vi "TelemetryServer.vi"() -> ()   [LabVIEW 2009]
uses:
  Api/TelemetryServer/TelemetryServer_Global.vi
  Instance           7 23Saved   TelemetryServer .vi
panel:
  in  "PROCESS":string="TELEMETRYSERVER"
  out "Counts":u32[](array[numeric])
  out "ID":u32
  in  "ServerName":string="RTC21Summit.Telemetry.Default"
  in  "Channels":string[](array[string])=["FringeTracker[0].CompleteControllerSet.ControllerData.ChannelData[0].CalibratedBinData[0]", "FringeTracker[0].CompleteControllerSet.ControllerData.DLPosition", "StarTracker[1].CompleteControllerSet.KatControllerData.Intensity", "StarTracker[1].CompleteControllerSet.KatControllerData.PeakIntensity", "StarTracker[1].CompleteControllerSet.KatControllerData.FsmX", "StarTracker[1].CompleteControllerSet.KatControllerData.FsmY", "StarTracker[1].CompleteControllerSet.KatControllerData.PointVectorX", "StarTracker[1].CompleteControllerSet.KatControllerData.PointVectorY", "StarTracker[2].CompleteControllerSet.KatControllerData.Intensity", "StarTracker[2].CompleteControllerSet.KatControllerData.PeakIntensity", "StarTracker[2].CompleteControllerSet.KatControllerData.FsmX", "StarTracker[2].CompleteControllerSet.KatControllerData.FsmY", "StarTracker[2].CompleteControllerSet.KatControllerData.PointVectorX", "StarTracker[2].CompleteControllerSet.KatControllerData.PointVectorY", "StarTracker[3].CompleteControllerSet.KatControllerData.Intensity", "StarTracker[4].CompleteControllerSet.KatControllerData.Intensity", "DelayLine[1].CompleteControllerSet.ControllerData.LaserPositionOPD"]
  out "Count":i32(knob)=17 scale=0.0..34.0
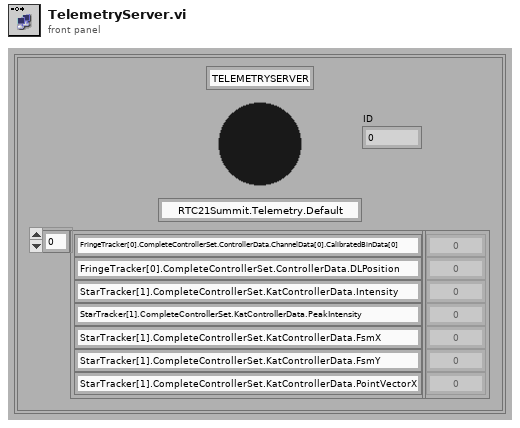
[diagram p1: front panel]
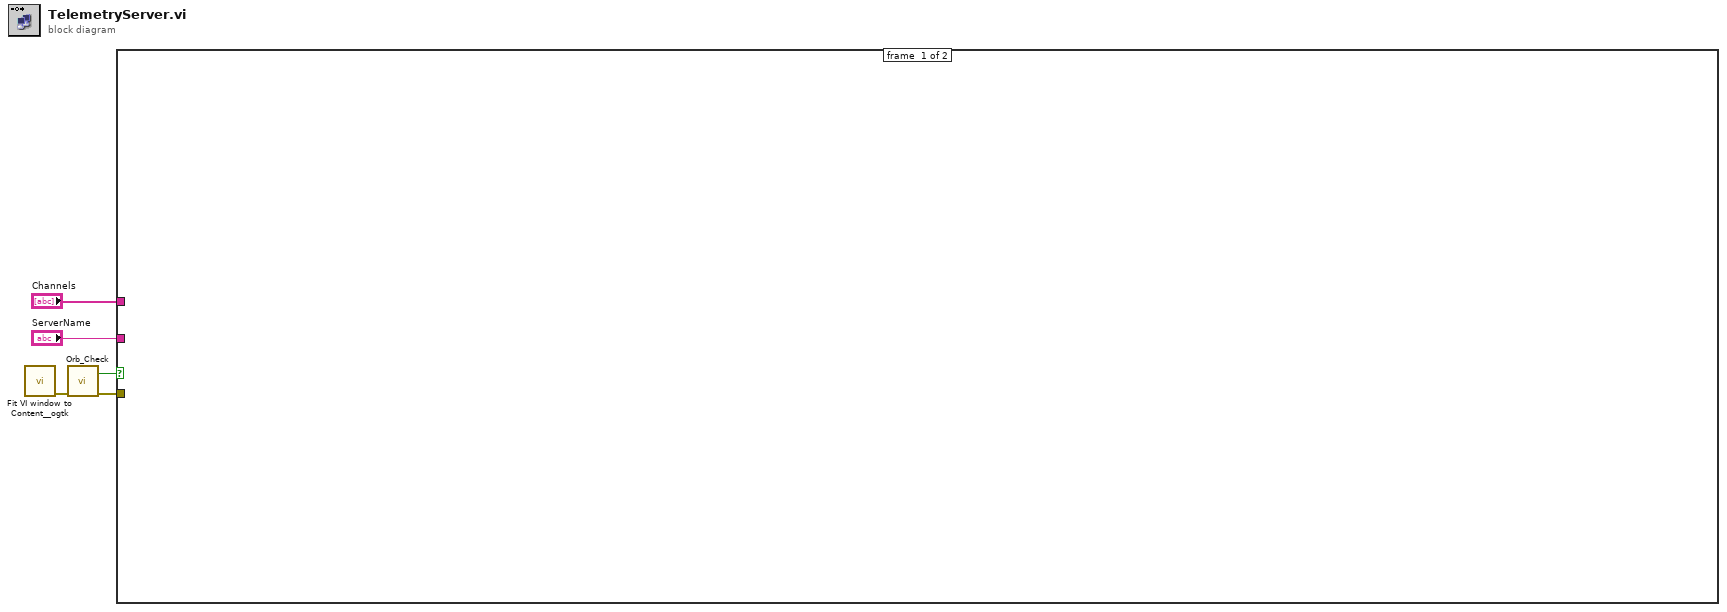
[diagram p0: block diagram]
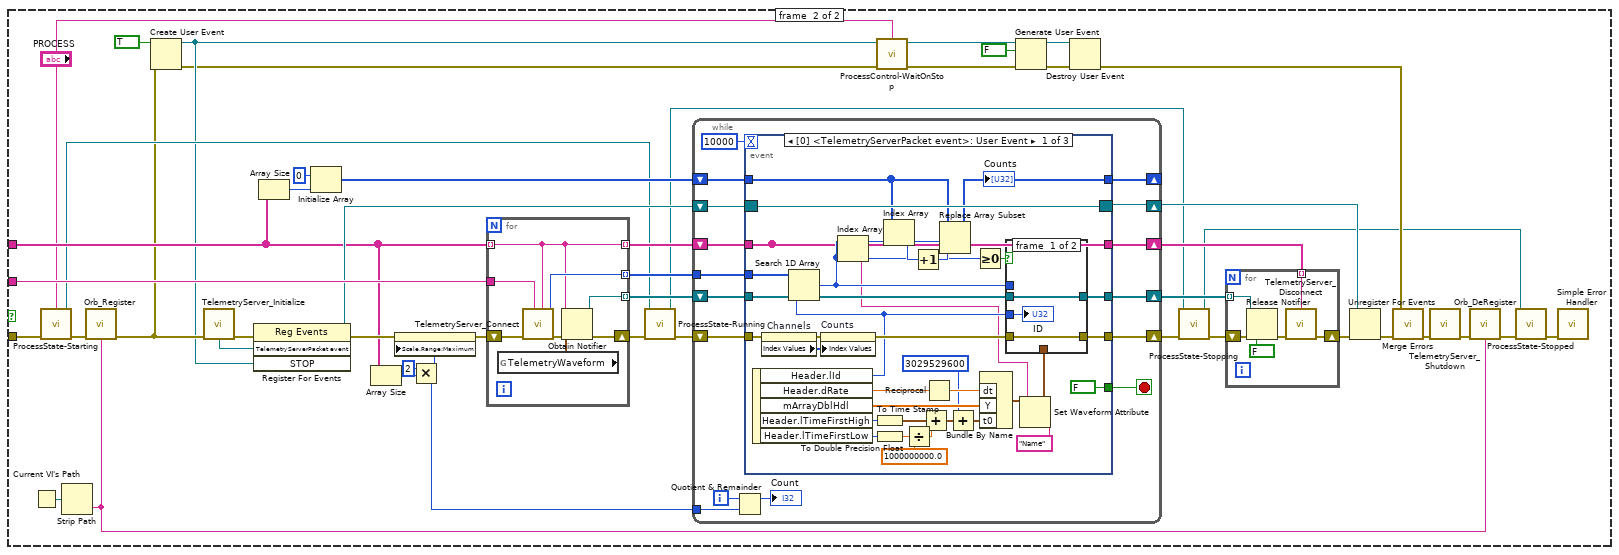
[diagram p2: hidden frame]
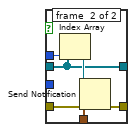
[diagram p3: hidden frame]
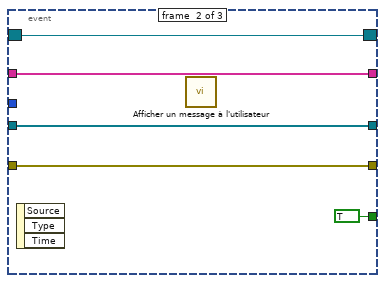
[diagram p4: hidden frame]
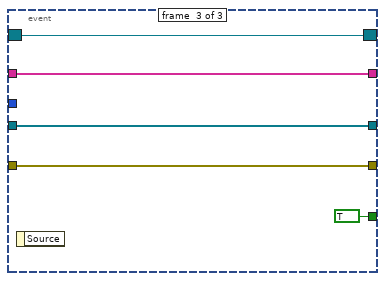
[diagram p5: hidden frame]
diagram:
  n1 = call <userlib>:"Fit VI window to Content__ogtk.vi"() -> ("error out"=w1:errorcluster)  [unwired: 3 in, 4 out]
  n2 = call "Orb_Check.vi"("error in (no error)"=w1) -> ("error out"=w5:errorcluster, "Orb Running ?"=w4:bool)  [unwired: 4 out]
  n3 = case shown="True" w4 {
    tunnel: w5 -> [_ w25]
    tunnel: "Channels" -> [_ w29]
    tunnel: "ServerName" -> [_ w37]
    frame #0 {
    }
    frame #1 {
      n4 = Current VI's Path() -> (path=w45:path)
      n5 = call "ProcessState-Starting.vi"("PROCESS"="PROCESS", "error in (no error)"=w25) -> ("ProcessStateNotifier"=w21:refnum<notifier>, "error in (no error)"=w24:errorcluster)  [unwired: 6 out]
      n6 = Strip Path(path=w45) -> (name=w39:string)  [unwired: 1 out]
      n7 = call "Orb_Register.vi"("error in (no error)"=w24, "Registering VI"=w39) -> ("error out"=w18:errorcluster)  [unwired: 5 out]
      n8 = Create User Event(user event datatype=TRUE ("STOP"), error in=w18) -> (user event=w17:refnum<user-event>, error out=w16:errorcluster)
      n9 = call "TelemetryServer_Initialize.vi"("error in (no error)"=w18) -> ("error out"=w51:errorcluster, "TelemetryServerPacket event"=w50:refnum<user-event>)  [unwired: 7 out]
      n10 = register-events(error in=w51, w50, w17) -> (reference out=w32:refnum<event-registration>, error out=w38:errorcluster)  [unwired: 1 in]
      n11 = Array Size(array=w29) -> (size(s)=w28:i32)
      n12 = Initialize Array(u32 0, w28) -> (w26:u32[])
      n13 = Array Size(array=w29) -> (size(s)=w43:i32)
      n14 = Multiply(x=2, y=w43) -> (x*y=w41:i32)
      n15 = property on="Count" class="Bouton rotatif (strict)"(error in=w38, "Scale.Range:Maximum"=w41) -> (error out=w44:errorcluster)  [unwired: 1 in, 1 out]
      n16 = for {
        tunnel: [w65] -> w49 mode=indexing
        shift-right: [w63] -> w23
        shift-left: w44 -> [w60]
        tunnel: [w62] -> w47 mode=indexing
        tunnel: [w58] -> w35 mode=indexing
        tunnel: w37 -> [w59]
        tunnel: w29 -> [w58] mode=indexing
        n17 = global read "TelemetryServer_Global.vi" "TelemetryWaveform"() -> (w61:waveform(dbl))
        n18 = call "TelemetryServer_Connect.vi"("Channel Name"=w58, "Server Name"=w59, "error in (no error)"=w60) -> ("error out"=w64:errorcluster, "Channel Id"=w65:u32)  [unwired: 1 in, 4 out]
        n19 = Obtain Notifier(name (unnamed)=w58, notification data type=w61, error in (no error)=w64) -> (notifier out=w62:refnum<notifier>, error out=w63:errorcluster)  [unwired: 1 in, 1 out]
      }
      n20 = call "ProcessState-Running.vi"("ProcessStateNotifier in"=w21, "error in (no error)"=w23) -> ("ProcessStateNotifier out"=w9:refnum<notifier>, "error out"=w22:errorcluster)  [unwired: 6 out]
      n21 = while {
        shift-right: [w81] -> w11
        shift-left: w22 -> [w80]
        tunnel: w49 -> [w77]
        shift-right: [w75] -> w46
        shift-left: w47 -> [w76]
        shift-right: [w78] -> w31
        shift-left: w32 -> [w79]
        tunnel: w41 -> [w67]
        shift-right: [w66] -> w34
        shift-left: w35 -> [w68]
        shift-right: [w69] -> _
        shift-left: w26 -> [w70]
        i -> [w73]
        stop <- w71 stop-if-true
        n22 = Quotient & Remainder(x=w73, y=w67) -> (x-y*floor(x/y)=→"Count":i32)  [unwired: 1 out]
        n23 = event shown="[0] <TelemetryServerPacket event>: User Event" {
          selector: w79 -> [w115 w129 w134]
          dyn-events: [w115 w129 w134] -> w78
          timeout: 10000 -> [_ _ _]
          tunnel: [w114 w127 w133] -> w81
          tunnel: [FALSE ("stop") TRUE ("stop") TRUE ("stop")] -> w71
          tunnel: w80 -> [w93 w127 w133]
          tunnel: w77 -> [w113 _ _]
          tunnel: w76 -> [w112 w128 w132]
          tunnel: [w109 w128 w132] -> w75
          tunnel: w70 -> [w99 _ _]
          tunnel: [w98 _ _] -> w69
          tunnel: w68 -> [w85 w125 w130]
          tunnel: [w85 w125 w130] -> w66
          event #0 {
            n24 = event-data() -> ("Header.lId"=w90:u32, "Header.dRate"=w107:dbl, "mArrayDblHdl"=w106:dbl[], "Header.lTimeFirstHigh"=w101:u32, "Header.lTimeFirstLow"=w100:u32)  [unwired: 1 out]
            n25 = property on="Channels" class="Tableau (strict)"(error in=w93) -> (error out=w95:errorcluster, "Index Values"=w94:u32[])  [unwired: 1 in, 1 out]
            n26 = Search 1D Array(1D array=w113, element=w90) -> (index of element=w91:i32)  [unwired: 1 out]
            n27 = property on="Counts" class="Tableau (strict)"(error in=w95, "Index Values"=w94) -> (error out=w92:errorcluster)  [unwired: 1 in, 1 out]
            n28 = Index Array(array=w85, index=w91) -> (element=w86:string)
            n29 = To Time Stamp(1:w101) -> (0:w103:timestamp)
            n30 = To Double Precision Float(number=w100) -> (double precision float=w105:dbl)
            n31 = Index Array(array=w99, index=w91) -> (element=w97:u32)
            n32 = Divide(x=w105, y=1000000000.0) -> (x/y=w102:dbl)
            n33 = Increment(x=w97) -> (x+1=w96:u32)
            n34 = Add(x=w103, y=w102) -> (x+y=w84:timestamp)
            n35 = Reciprocal(x=w107) -> (1/x=w108:dbl)
            n36 = Replace Array Subset(array=w99, new element=w96, index=w91) -> (w98:u32[])
            "Counts" <- w98
            n37 = Add(x=w84, y=i64 3029529600) -> (x+y=w83:timestamp)
            n38 = Greater Or Equal To 0?(x=w91) -> (x >= 0?=w110:bool)
            n39 = Bundle By Name("dt"=w108, "Y"=w106, "t0"=w83) -> (w89:waveform(dbl))  [unwired: 1 out]
            n40 = Set Waveform Attribute(5:w86, 6:"Name" ("nom"), 7:w89) -> (3:w88:waveform(dbl))  [unwired: 1 in, 2 out]
            n41 = case shown="True" w110 {
              tunnel: w92 -> [w117 w124]
              tunnel: [w117 w123] -> w114
              tunnel: w88 -> [_ w122]
              tunnel: w112 -> [w118 w119]
              tunnel: w91 -> [_ w120]
              tunnel: [w118 w119] -> w109
              tunnel: w90 -> [w116 _]
              frame #0 {
                "ID" <- w116
              }
              frame #1 {
                n42 = Index Array(array=w119, index=w120) -> (element=w121:refnum<notifier>)
                n43 = Send Notification(notification=w122, notifier=w121, error in (no error)=w124) -> (error out=w123:errorcluster)  [unwired: 1 out]
              }
            }
          }
          event #1 {
            n44 = event-data() -> ()  [unwired: 4 out]
            n45 = call "Afficher un message à l'utilisateur"() -> ()  [unwired: 3 in, 9 out]
          }
          event #2 {
            n46 = event-data() -> ()  [unwired: 2 out]
          }
        }
      }
      n47 = call "ProcessControl-WaitOnStop.vi"("PROCESS"="PROCESS", "error out"=w16) -> ("error in"=w19:errorcluster)  [unwired: 7 out]
      n48 = Generate User Event(user event=w17, event data cluster=FALSE ("données d'événement"), error in=w19) -> (user event out=w30:refnum<user-event>, error out=w15:errorcluster)
      n49 = Destroy User Event(user event=w30, error in=w15) -> (error out=w12:errorcluster)
      n50 = call "ProcessState-Stopping.vi"("ProcessStateNotifier in"=w9, "error in (no error)"=w11) -> ("ProcessStateNotifier out"=w7:refnum<notifier>, "error out"=w10:errorcluster)  [unwired: 6 out]
      n51 = for {
        shift-right: [w57] -> w48
        shift-left: w10 -> [w55]
        tunnel: w34 -> [w56] mode=indexing
        tunnel: w46 -> [w52] mode=indexing
        n52 = Release Notifier(notifier=w52, force destroy? (F)=FALSE ("forcer la destruction ? (F)"), error in (no error)=w55) -> (error out=w54:errorcluster)  [unwired: 2 out]
        n53 = call "TelemetryServer_Disconnect.vi"("Channel Name"=w56, "error in (no error)"=w54) -> ("error out"=w57:errorcluster)  [unwired: 7 out]
      }
      n54 = Unregister For Events(event registration refnum=w31, error in=w48) -> (error out=w13:errorcluster)
      n55 = call <vilib>:"Merge Errors.vi"("error in 3 (no error)"=w13, "error in 1 (no error)"=w12) -> ("error out"=w14:errorcluster)  [unwired: 2 in, 3 out]
      n56 = call "TelemetryServer_Shutdown.vi"("error in (no error)"=w14) -> ("error out"=w40:errorcluster)  [unwired: 8 out]
      n57 = call "Orb_DeRegister.vi"("error in (no error)"=w40, "De-registering VI"=w39) -> ("error out"=w8:errorcluster)  [unwired: 5 out]
      n58 = call "ProcessState-Stopped.vi"("ProcessStateNotifier in"=w7, "error in (no error)"=w8) -> ("error out"=w6:errorcluster)  [unwired: 7 out]
      n59 = call <vilib>:"Simple Error Handler.vi"("error in (no error)"=w6) -> ()  [unwired: 1 in, 8 out]
    }
  }
